vi "TextFit_Build Character Cluster array.vi"(8 "Error":errorcluster, 11 "String":string) -> (0 "Error Out":errorcluster, 3 "Character Array Out":T1[](array[typedef]))   [LabVIEW 2014]
doc: "Builds a character cluster array from an input string"
uses:
  Controls/Cluster/Cluster_Character Size and Priority Data.ctl
  Controls/String_Picture/String Char Normal.ctl
  Controls/Enum/ENUM_Font Size Select.ctl
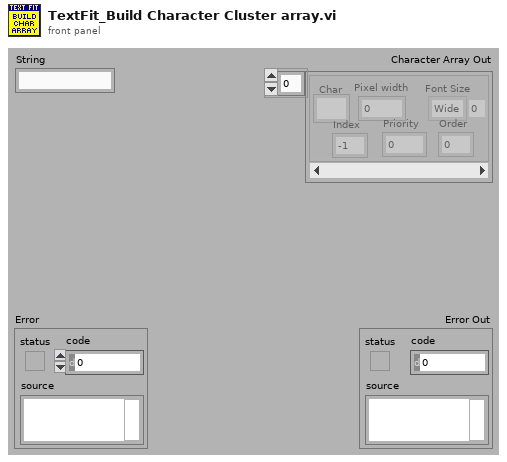
[diagram p1: front panel]
types:
  T1 = typedef "Cluster_Character Size and Priority Data.ctl" = cluster{"Char":T2, "Font Size":T3, "Pixel width":i32, "Priority":i32, "Order":i32, "Index":i32}
  T2 = typedef "String Char Normal.ctl" = string
  T3 = typedef "ENUM_Font Size Select.ctl" = enum16{"Wide", "Med", "Thin"}
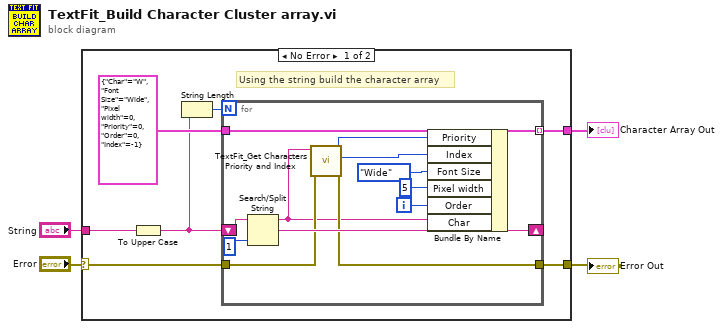
[diagram p0: block diagram]
diagram:
  n1 = case shown="No Error" "Error" {
    selector: "Error" -> [w5 w25]
    tunnel: [w11 w25] -> w4
    tunnel: [w10 _] -> w3
    tunnel: "String" -> [w7 _]
    frame No Error {
      # "Using the string build the character array"
      n2 = To Upper Case(1:w7) -> (0:w8:string)
      n3 = String Length(string=w8) -> (length=w6:i32)
      n4 = for {
        N: w6 -> [_]
        shift-right: [w17] -> _
        shift-left: w8 -> [w18]
        tunnel: T1 {"Char"="W", "Font Size"=enum."Wide", "Pixel width"=0, "Priority"=0, "Order"=0, "Index"=-1} ("Cluster") -> [w23]
        tunnel: [w22] -> w10 mode=indexing
        tunnel: w5 -> [w14]
        tunnel: [w13] -> w11
        i -> [w19]
        n5 = Search/Split String(string=w18, offset (0)=1) -> (substring before match=w12:string, match + rest of string=w17:string)  [unwired: 1 in, 1 out]
        n6 = call "TextFit_Get Characters Priority and Index.vi"("Error"=w14, "Char"=w12) -> ("Error Out"=w13:errorcluster, "Index Out"=w16:i32, "Priority Out"=w15:i32)  [unwired: 7 in]
        n7 = Bundle By Name(cluster=w23, "Priority"=w15, "Index"=w16, "Font Size"=ENUM_Font_Size_Select."Wide" ("Font Size Select"), "Pixel width"=5 ("Pixel with"), "Order"=w19, "Char"=w12) -> (w22:T1)
      }
    }
    frame Error {
    }
  }
  "Error Out" <- w4
  "Character Array Out" <- w3
